vi "Lvi Trigger Properties.vi"(0 "TaskRef":i32, 11 "error in (no error)":errorcluster) -> (1 "SupSvPosExtTTL":bool, 2 "SupSoftware":bool, 3 "SupPosExtTTL":bool, 4 "TaskRef out":i32, 6 "SupDigitalEvent":bool, 8 "SupNegExtTTL":bool, 10 "SupNegThresh":bool, 12 "function return":u32(ring), 13 "SupSvNegExtTTL":bool, 14 "SupPosThresh":bool, 15 "error out":errorcluster)   [LabVIEW 2022 SP3, in "DtLvLink.lvlib"]
doc: "Calls directly into the entry points of the DLL of the Data Acq SDK to return information about the trigger source of the device. This VI is used by the higher-level VI, DtOLTriggerSource."
uses:
  DtLvLink.lvlib
  <userlib>/LV-Link3/DtLvLink_64.dll
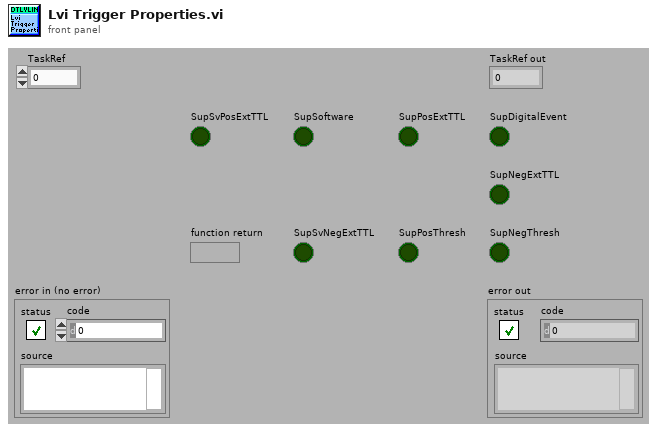
[diagram p1: front panel]
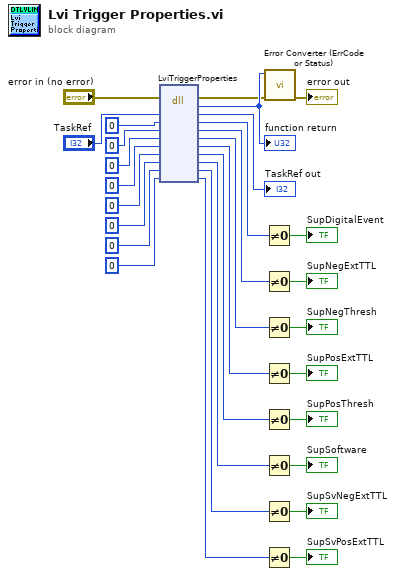
[diagram p0: block diagram]
diagram:
  n1 = dll-call lib="C:/Program Files/National Instruments/LabVIEW 2022/user.lib/LV-Link3/DtLvLink_64.*" fn="LviTriggerProperties"(error in="error in (no error)", "TaskRef"="TaskRef", "SupDigitalEvent"=u8 0, "SupNegExtTTL"=u8 0, "SupNegThresh"=u8 0, "SupPosExtTTL"=u8 0, "SupPosThresh"=u8 0, "SupSoftware"=u8 0, "SupSvNegExtTTL"=u8 0, "SupSvPosExtTTL"=u8 0) -> (error out=w2:errorcluster, w30:u32, "TaskRef"=→"TaskRef out":i32, "SupDigitalEvent"=w25:u8, "SupNegExtTTL"=w22:u8, "SupNegThresh"=w19:u8, "SupPosExtTTL"=w16:u8, "SupPosThresh"=w13:u8, "SupSoftware"=w10:u8, "SupSvNegExtTTL"=w7:u8, "SupSvPosExtTTL"=w4:u8)  [unwired: 2 in, 1 out]
  "function return" <- w30
  n2 = Not Equal To 0?(x=w25) -> (x != 0?=→"SupDigitalEvent":bool)
  n3 = Not Equal To 0?(x=w22) -> (x != 0?=→"SupNegExtTTL":bool)
  n4 = Not Equal To 0?(x=w19) -> (x != 0?=→"SupNegThresh":bool)
  n5 = Not Equal To 0?(x=w16) -> (x != 0?=→"SupPosExtTTL":bool)
  n6 = Not Equal To 0?(x=w13) -> (x != 0?=→"SupPosThresh":bool)
  n7 = Not Equal To 0?(x=w10) -> (x != 0?=→"SupSoftware":bool)
  n8 = Not Equal To 0?(x=w7) -> (x != 0?=→"SupSvNegExtTTL":bool)
  n9 = Not Equal To 0?(x=w4) -> (x != 0?=→"SupSvPosExtTTL":bool)
  n10 = call "Error Converter (ErrCode or Status).vi"("error in (no error)"=w2, "error code"=w30) -> ("error out"=→"error out":errorcluster)  [unwired: 9 in]
